vi "Set IConfigure.vi"(8 "Error In":errorcluster, 10 "IConfigure":refnum<class "IConfigure.lvclass">, 11 "reference in":refnum<class "NI9862.lvclass">) -> (0 "Error Out":errorcluster, 3 "reference out":refnum<class "NI9862.lvclass">)   [LabVIEW 2024, in "NI9862.lvclass"]
uses:
  NI9862.lvclass
  NI9862.lvclass/NI9862.ctl
  Source/Interfaces/IConfigure/IConfigure.lvclass
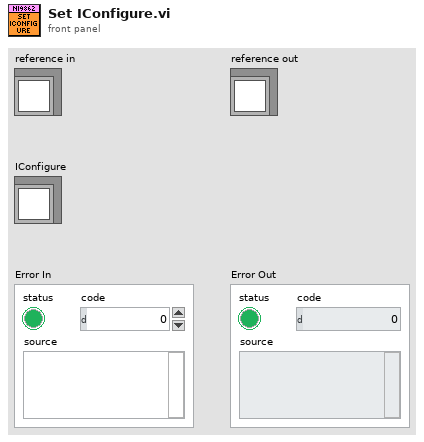
[diagram p1: front panel]
types:
  T1 = typedef "NI9862.lvclass/ObjectAttributes.ctl" = cluster{"IConfigure":refnum<class "IConfigure.lvclass">}
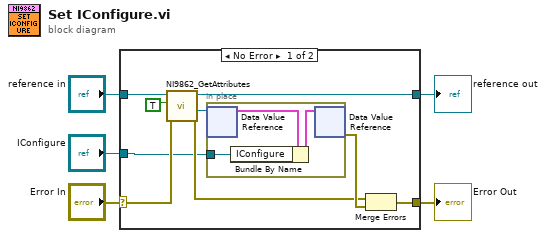
[diagram p0: block diagram]
diagram:
  n1 = case shown="No Error" "Error In" {
    selector: "Error In" -> [w12 w19]
    tunnel: [w7 w19] -> w4
    tunnel: [w13 w18] -> w2
    tunnel: "reference in" -> [w14 w18]
    tunnel: "IConfigure" -> [w6 _]
    frame No Error {
      n2 = call "NI9862_GetAttributes.vi"("Error In"=w12, "OnlyGetDvrReference(False)"=TRUE, "NI9862 in"=w14) -> ("Error Out"=w8:errorcluster, "DataRef"=w9:refnum<data-value>, "NI9862 out"=w13:refnum<class "NI9862.lvclass">)  [unwired: 5 in, 1 out]
      n3 = in-place {
        in-place-border: w6 -> [w15]
        n4 = in-place-dvr #1(w9) -> (w16:T1)  [unwired: 1 out]
        n5 = Bundle By Name(cluster=w16, "IConfigure"=w15) -> (w17:T1)
        n6 = in-place-dvr #1(w17) -> (w10:errorcluster)  [unwired: 1 out]
      }
      n7 = Merge Errors(w8, w10) -> (w7:errorcluster)
    }
    frame Error {
    }
  }
  "Error Out" <- w4
  "reference out" <- w2
